vi "test12.1-SyncMessage_Event.vi"(8 "error in (no error)":errorcluster, 11 "TestCase in":refnum<class "testcase-CSMGlobalLog.lvclass">) -> (0 "error out":errorcluster, 3 "TestCase out":refnum<class "testcase-CSMGlobalLog.lvclass">)   [LabVIEW 2017, in "testcase-CSMGlobalLog.lvclass"]
uses:
  testcase-CSMGlobalLog.lvclass
  testcase-CSMGlobalLog.lvclass/testcase-CSMGlobalLog.ctl
  src/user.lib/_NEVSTOP/Communicable State Machine(CSM)/_Support/Typedef/_CSM_GlobalLog_MSG.ctl
  src/user.lib/_NEVSTOP/Communicable State Machine(CSM)/_Support/Typedef/_CSM_Response Source Message.ctl
  src/user.lib/_NEVSTOP/Communicable State Machine(CSM)/_Support/Typedef/_CSM_GlobalLog_MSG_TYPE.ctl
  c0dc643a-0362-49fc-99f4-5251266ba5a0.vi
  src/user.lib/_NEVSTOP/Communicable State Machine(CSM)/_Support/GlobalEvent/GEvt-Generate with Rule Check.vi
  src/user.lib/_NEVSTOP/Communicable State Machine(CSM)/AdvanceAPI/CSM - Convert Error to Argument.vi
  src/user.lib/_NEVSTOP/Communicable State Machine(CSM)/_Support/GlobalEvent/Cache-GEvt Filter Object.vi
  src/user.lib/_NEVSTOP/Communicable State Machine(CSM)/_Support/GlobalEvent/Cache-GEvt Refs.vi
  src/user.lib/_NEVSTOP/Communicable State Machine(CSM)/AdvanceAPI/CSM - Make String Arguments Safe.vi
  src/user.lib/_NEVSTOP/Communicable State Machine(CSM)/_Support/GlobalEvent/GEvt-Convert Filter Rules - v1.2.vi
  src/user.lib/_NEVSTOP/Communicable State Machine(CSM)/_Support/ChangeFlag/FlagInstance-GEvt Filter.vi
  src/user.lib/_NEVSTOP/Communicable State Machine(CSM)/_Support/ChangeFlag/FlagInstance-GEvt Refs.vi
  src/user.lib/_NEVSTOP/Communicable State Machine(CSM)/AdvanceAPI/CSM - Keywords.vi
  src/user.lib/_NEVSTOP/Communicable State Machine(CSM)/_Support/ChangeFlag/ChangeFlag-Read.vi
  src/user.lib/_NEVSTOP/Communicable State Machine(CSM)/_Support/ChangeFlag/ChangeFlagDB.vi
  src/user.lib/_NEVSTOP/Communicable State Machine(CSM)/_Support/GlobalEvent/FGV-GlobalEventRef(lvlibp).vi
  src/user.lib/_NEVSTOP/Communicable State Machine(CSM)/_Support/GlobalEvent/FGV-GlobalEventQueues(lvlibp).vi
  src/user.lib/_NEVSTOP/Communicable State Machine(CSM)/_Support/GlobalEvent/GEvt-Valid Subscribers.vi
  src/user.lib/_NEVSTOP/Communicable State Machine(CSM)/_Support/GlobalEvent/FGV-GEvt Filter Rules(lvlibp).vi
  src/user.lib/_NEVSTOP/Communicable State Machine(CSM)/_Support/GlobalEvent/LogFilter/SettingVIs/Set Global CSM Filter.vi
  src/user.lib/_NEVSTOP/Communicable State Machine(CSM)/_Support/GlobalEvent/LogFilter/SettingVIs/Set Global LogType Filter.vi
  src/user.lib/_NEVSTOP/Communicable State Machine(CSM)/_Support/GlobalEvent/LogFilter/SettingVIs/Set Global State Filter.vi
  src/user.lib/_NEVSTOP/Communicable State Machine(CSM)/_Support/GlobalEvent/LogFilter/SettingVIs/Set Global Broadcast Filter.vi
  src/user.lib/_NEVSTOP/Communicable State Machine(CSM)/_Support/GlobalEvent/LogFilter/SettingVIs/Set Global UserLog Filter.vi
  src/user.lib/_NEVSTOP/Communicable State Machine(CSM)/_Support/GlobalEvent/LogFilter/SettingVIs/Set CSM LogType Filter.vi
  src/user.lib/_NEVSTOP/Communicable State Machine(CSM)/_Support/GlobalEvent/LogFilter/SettingVIs/Set CSM State Filter.vi
  src/user.lib/_NEVSTOP/Communicable State Machine(CSM)/_Support/GlobalEvent/LogFilter/SettingVIs/Set Global StateType Filter.vi
  src/user.lib/_NEVSTOP/Communicable State Machine(CSM)/_Support/GlobalEvent/LogFilter/SettingVIs/Set CSM StateType Filter.vi
  src/user.lib/_NEVSTOP/Communicable State Machine(CSM)/_Support/GlobalEvent/LogFilter/SettingVIs/Set CSM Broadcast Filter.vi
  src/user.lib/_NEVSTOP/Communicable State Machine(CSM)/_Support/GlobalEvent/LogFilter/SettingVIs/Set CSM UserLog Filter.vi
  src/user.lib/_NEVSTOP/Communicable State Machine(CSM)/_Support/GlobalEvent/LogFilter/SettingVIs/Set Periodic Log Filter.vi
  src/user.lib/_NEVSTOP/Communicable State Machine(CSM)/_Support/GlobalEvent/LogFilter/LogFilter - Check.vi
  src/user.lib/_NEVSTOP/Communicable State Machine(CSM)/_Support/GlobalEvent/LogFilter/LogFilter.lvclass
  <vilib>/addons/_JKI Toolkits/VI Tester/TestCase.llb/TestCase.lvclass
  src/user.lib/_NEVSTOP/Communicable State Machine(CSM)/Communicable State Machine.lvlib
  C:/Program Files (x86)/National Instruments/LabVIEW 2017/vi.lib/addons/_JKI Toolkits/VI Tester/TestCase.llb/TestCase.lvclass
panel:
  out "String cache each loop":string
  out "LoopCount":i32
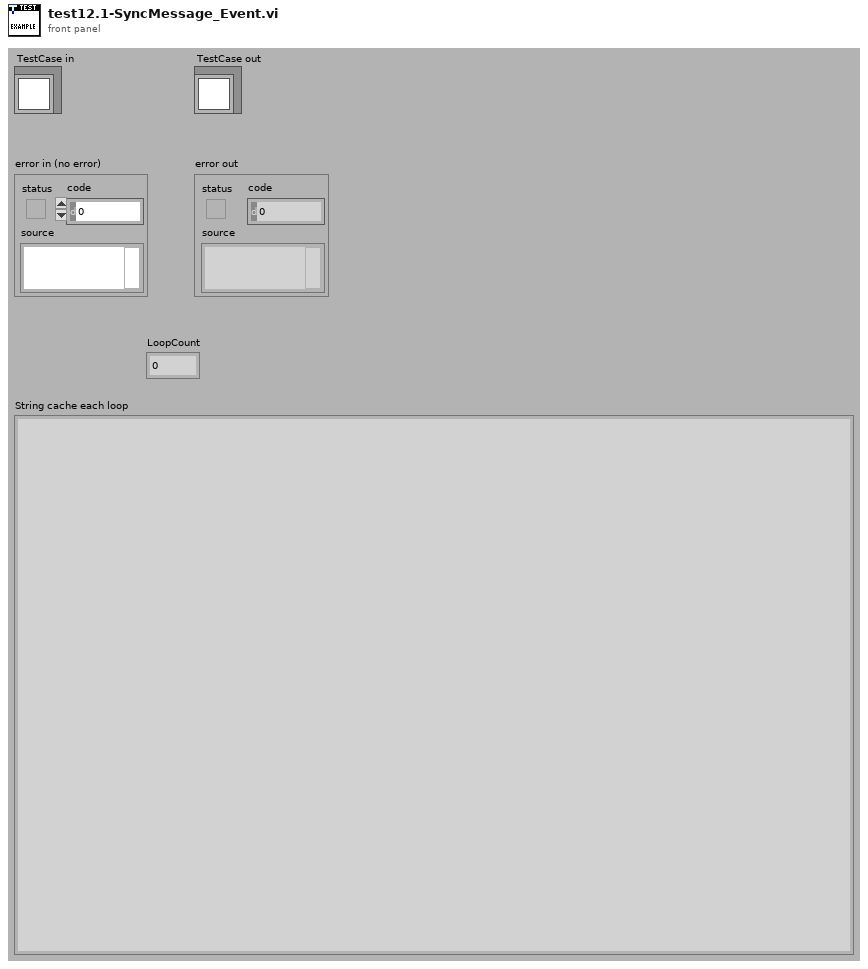
[diagram p1: front panel]
types:
  T1 = typedef "Communicable State Machine.lvlib/_CSM_GlobalLog_MSG.ctl" = cluster{"Name (\"\" to Use UUID)":string, "Current State":string, "Arguments":string, "Source Message":T2, "Source Module":string, "Complete(T)/Start(F)":bool, "LogType":T3, "Time Stamp":timestamp}
  T2 = typedef "Communicable State Machine.lvlib/_CSM_Response Source Message.ctl" = cluster{"‘State":string, "’Arguments":string, "’Error":errorcluster}
  T3 = typedef "Communicable State Machine.lvlib/_CSM_GlobalLog_MSG_TYPE.ctl" = enum16{"User Log", "State Change", "Status", "Interrupt", "Register", "Unregister", "Error Log", "Module Created", "Module Destroyed", "Async Message", "No-Rep Async Message", "Sync Message", "AsyncMsg Complete", "SyncMsg Complete"}
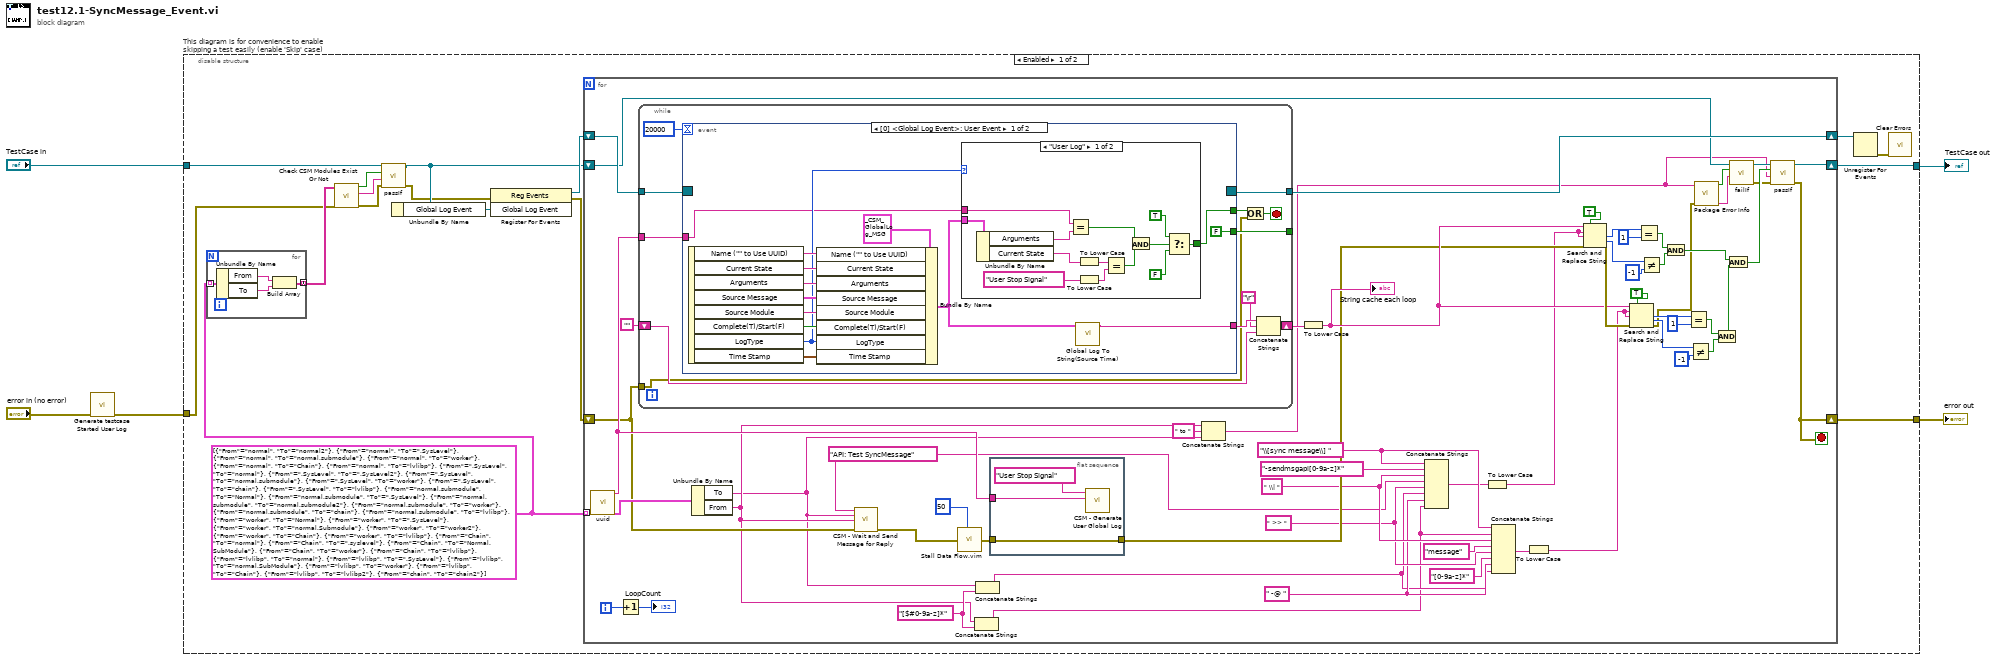
[diagram p0: block diagram]
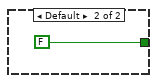
[diagram p2: hidden frame]
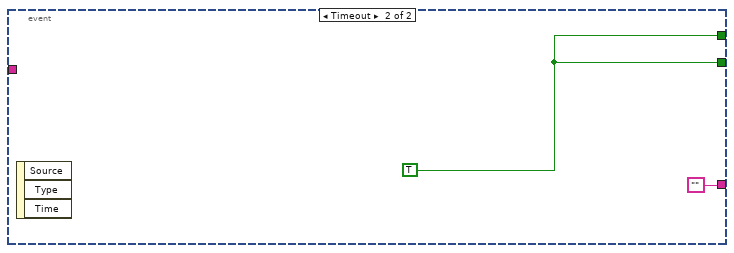
[diagram p3: hidden frame]
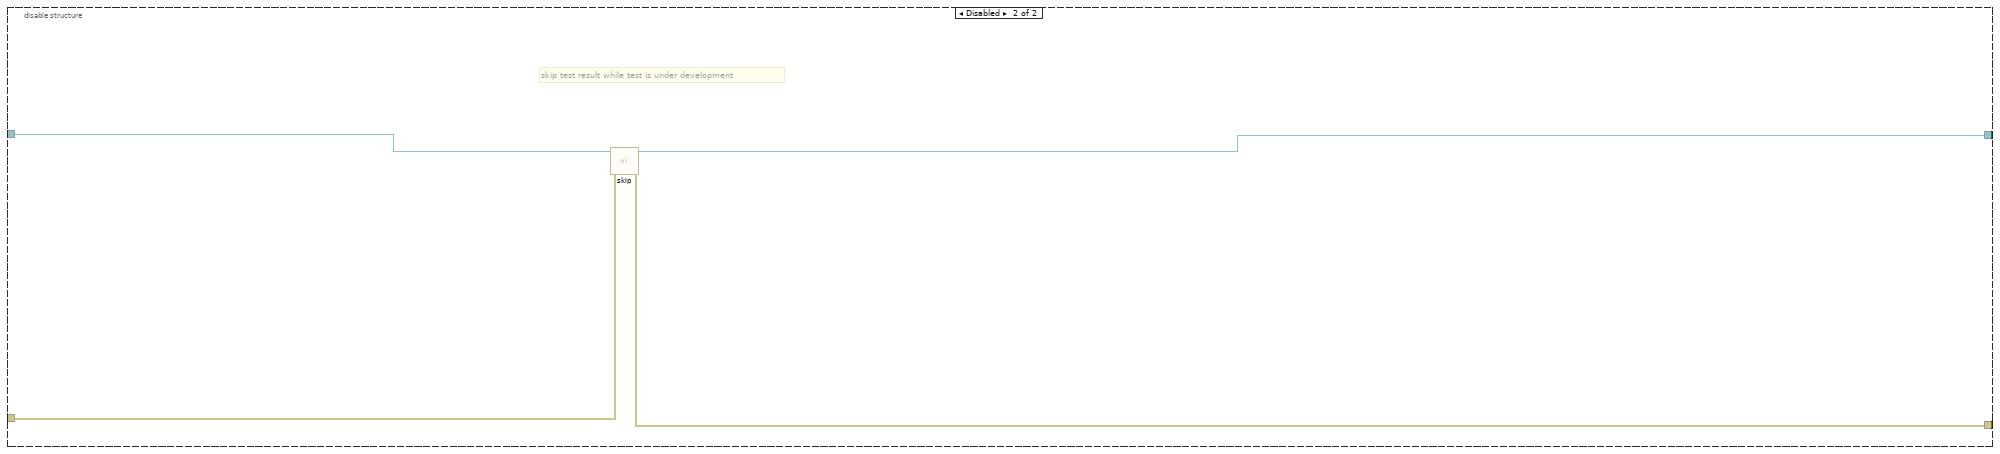
[diagram p4: hidden frame]
diagram:
  n1 = call "Generate testcase Started User Log.vi"("Error In"="error in (no error)") -> ("error out"=w1:errorcluster)  [unwired: 10 in]
  n2 = disable-structure "This diagram is for convenience to enable skipping a test easily (enable 'Skip' case)" shown="Enabled" {
    disable-tunnel: "TestCase in" -> [w9 w133]
    disable-tunnel: [w17 w131] -> w2
    disable-tunnel: [w16 w132] -> w4
    disable-tunnel: w1 -> [w10 w130]
    frame Enabled {
      w11 = cluster{"From":string, "To":string}[] [{"From"="normal", "To"="normal2"}, {"From"="normal", "To"=".SysLevel"}, {"From"="normal", "To"="normal.submodule"}, {"From"="normal", "To"="worker"}, {"From"="normal", "To"="Chain"}, {"From"="normal", "To"="lvlibp"}, {"From"=".SysLevel", "To"="normal"}, {"From"=".SysLevel", "To"=".SysLevel2"}, {"From"=".SysLevel", "To"="normal.submodule"}, {"From"=".SysLevel", "To"="worker"}, {"From"=".SysLevel", "To"="chain"}, {"From"=".SysLevel", "To"="lvlibp"}, {"From"="normal.submodule", "To"="Normal"}, {"From"="normal.submodule", "To"=".SysLevel"}, {"From"="normal.submodule", "To"="normal.submodule2"}, {"From"="normal.submodule", "To"="worker"}, {"From"="normal.submodule", "To"="chain"}, {"From"="normal.submodule", "To"="lvlibp"}, {"From"="worker", "To"="Normal"}, {"From"="worker", "To"=".SysLevel"}, {"From"="worker", "To"="normal.Submodule"}, {"From"="worker", "To"="worker2"}, {"From"="worker", "To"="Chain"}, {"From"="worker", "To"="lvlibp"}, {"From"="Chain", "To"="normal"}, {"From"="Chain", "To"=".syslevel"}, {"From"="Chain", "To"="Normal.SubModule"}, {"From"="Chain", "To"="worker"}, {"From"="Chain", "To"="lvlibp"}, {"From"="lvlibp", "To"="normal"}, {"From"="lvlibp", "To"=".SysLevel"}, {"From"="lvlibp", "To"="normal.SubModule"}, {"From"="lvlibp", "To"="worker"}, {"From"="lvlibp", "To"="Chain"}, {"From"="lvlibp", "To"="lvlibp2"}, {"From"="chain", "To"="chain2"}]
      n3 = for {
        tunnel: w11 -> [w25] mode=indexing
        tunnel: [w22] -> w13 mode=concatenating
        n4 = Unbundle By Name(w25) -> ("From"=w24:string, "To"=w23:string)
        n5 = Build Array(w24, w23) -> (w22:string[])
      }
      n6 = call "Check CSM Modules Exist Or Not.vi"("error in"=w10, "CSM names in"=w13) -> ("error out"=w15:errorcluster, "Debug string"=w14:string, "All Modules Exist?"=w12:bool)  [unwired: 7 in]
      n7 = call-dynamic "passIf.vi"("error in (no error)"=w15, "message (\"\")"=w14, "pass"=w12, "TestCase in"=w9) -> ("error out"=w7:errorcluster, "TestCase out"=w8:refnum<class "testcase-CSMGlobalLog.lvclass">)  [unwired: 6 in]
      n8 = Unbundle By Name(w8) -> ("Global Log Event"=w21:refnum<user-event>)
      n9 = register-events(error in=w7, w21) -> (reference out=w20:refnum<event-registration>, error out=w18:errorcluster)  [unwired: 1 in]
      n10 = for {
        shift-right: [w83] -> w19
        shift-left: w20 -> [w84]
        shift-right: [w80] -> w16
        shift-left: w18 -> [w36]
        tunnel: w11 -> [w61] mode=indexing
        shift-right: [w82] -> w17
        shift-left: w8 -> [w34]
        i -> [w58]
        stop <- w80 stop-if-true
        w39 = "[$#0-9a-z]*" ("string")
        w45 = " -@ "
        w47 = " >> "
        w49 = " \\| "
        w50 = "\\[sync message\\] "
        w42 = "API: Test SyncMessage" ("State")
        n11 = call "uuid.vi"() -> ("UUID"=w59:string)  [unwired: 11 in]
        n12 = Increment(x=w58) -> (x+1=→"LoopCount":i32)
        n13 = while {
          tunnel: w84 -> [w99]
          tunnel: [w98] -> w83
          shift-right: [w91] -> w52
          shift-left: "" -> [w94]
          tunnel: w59 -> [w96]
          tunnel: [w95] -> _
          tunnel: w36 -> [w88]
          stop <- w90 stop-if-true
          n14 = event shown="[0] <Global Log Event>: User Event" {
            selector: w99 -> [_ _]
            dyn-events: [_ _] -> w98
            timeout: 20000 -> [_ _]
            tunnel: [w100 ""] -> w93
            tunnel: [w102 w129] -> w89
            tunnel: w96 -> [w103 _]
            tunnel: [FALSE ("Stop") w129] -> w95
            event User Event {
              n15 = event-data() -> ("Name (\"\" to Use UUID)"=w112:string, "Current State"=w111:string, "Arguments"=w110:string, "Source Message"=w109:T2, "Source Module"=w108:string, "Complete(T)/Start(F)"=w107:bool, "LogType"=w104:T3, "Time Stamp"=w106:timestamp)  [unwired: 1 in]
              n16 = Bundle By Name(cluster=T1 {"Name (\"\" to Use UUID)"="", "Current State"="", "Arguments"="", "Source Message"={"‘State"="", "’Arguments"="", "’Error"={"status"=FALSE, "code"=0, "source"=""}}, "Source Module"="", "Complete(T)/Start(F)"=FALSE, "LogType"=enum."State Change", "Time Stamp"=timestamp(0 s since 1904-01-01)} ("Cross CSM Data"), "Name (\"\" to Use UUID)"=w112, "Current State"=w111, "Arguments"=w110, "Source Message"=w109, "Source Module"=w108, "Complete(T)/Start(F)"=w107, "LogType"=w104, "Time Stamp"=w106) -> (w101:T1)
              n17 = case shown="\"User Log\"" w104 {
                tunnel: w101 -> [w126 _]
                tunnel: w103 -> [w125 _]
                tunnel: [w114 FALSE] -> w102
                frame "User Log" {
                  n18 = Unbundle By Name(w126) -> ("Arguments"=w124:string, "Current State"=w123:string)
                  n19 = Equal?(x=w125, y=w124) -> (x = y?=w118:bool)
                  n20 = To Lower Case(string=w123) -> (all lower case string=w122:string)
                  n21 = To Lower Case(string="User Stop Signal" ("Log")) -> (all lower case string=w120:string)
                  n22 = Equal?(x=w122, y=w120) -> (x = y?=w119:bool)
                  n23 = And(x=w118, y=w119) -> (x .and. y?=w117:bool)
                  n24 = Select(t=TRUE, s=w117, f=FALSE) -> (s? t:f=w114:bool)
                }
                frame Default {
                }
              }
              n25 = call "Global Log To String(Source Time).vi"("Log"=w101) -> ("Log String"=w100:string)  [unwired: 9 in]
            }
            event Timeout {
              w129 = TRUE ("Stop")
              n26 = event-data() -> ()  [unwired: 1 in, 3 out]
            }
          }
          n27 = Or(x=w89, y=w88) -> (x .or. y?=w90:bool)
          n28 = Concatenate Strings(w93, "\r", w94) -> (w91:string)
        }
        n29 = Unbundle By Name(w61) -> ("To"=w28:string, "From"=w29:string)
        n30 = call "CSM - Wait and Send Message for Reply.vi"("State"=w42, "Arguments (\"\")"=w28, "Target Module"=w29, "Error In (No Error)"=w36) -> ("error out"=w55:errorcluster)  [unwired: 8 in, 3 out]
        n31 = call "Stall Data Flow.vim"("value in"=w55, "milliseconds to wait"=u32 50) -> ("value out"=w60:errorcluster)  [unwired: 1 out]
        n32 = Concatenate Strings(w29, w39) -> (w37:string)
        n33 = Concatenate Strings(w28, w39) -> (w38:string)
        n34 = flat-sequence {
          tunnel: w59 -> [w86]
          tunnel: w60 -> [w85]
          tunnel: [w85] -> w53
          frame #0 {
            n35 = call "CSM - Generate User Global Log.vi"("Arguments"=w86, "Log"="User Stop Signal") -> ()  [unwired: 9 in, 1 out]
          }
        }
        n36 = Concatenate Strings(w29, " to " ("string"), w28) -> (w26:string)
        n37 = To Lower Case(string=w52) -> (all lower case string=w54:string)
        "String cache each loop" <- w54
        n38 = Concatenate Strings(w50, "-sendmsgapi[0-9a-z]*", w49, w42, w47, w38, w45, w37) -> (w44:string)
        n39 = To Lower Case(string=w44) -> (all lower case string=w41:string)
        n40 = Concatenate Strings(w50, w37, w49, "message", w47, "[0-9a-z]*", w45, w38) -> (w43:string)
        n41 = To Lower Case(string=w43) -> (all lower case string=w40:string)
        n42 = Search and Replace String(replace all?=TRUE ("replace all? (F)"), input string=w54, search string=w41, replace string=w41, error in=w53) -> (number of replacements=w69:i32, offset past replacement=w70:i32, error out=w77:errorcluster)  [unwired: 3 in, 1 out]
        n43 = Search and Replace String(replace all?=TRUE ("replace all? (F)"), input string=w54, search string=w40, replace string=w40, error in=w77) -> (number of replacements=w76:i32, offset past replacement=w75:i32, error out=w30:errorcluster)  [unwired: 3 in, 1 out]
        n44 = Equal?(x=w69, y=1) -> (x = y?=w71:bool)
        n45 = Not Equal?(x=w70, y=-1) -> (x != y?=w72:bool)
        n46 = And(x=w71, y=w72) -> (x .and. y?=w79:bool)
        n47 = Equal?(x=w76, y=1) -> (x = y?=w74:bool)
        n48 = Not Equal?(x=w75, y=-1) -> (x != y?=w73:bool)
        n49 = call "Package Error Info.vi"("error in"=w30, "String in"=w26) -> ("packed error info out"=w31:string, "error status"=w35:bool)  [unwired: 8 in]
        n50 = And(x=w74, y=w73) -> (x .and. y?=w78:bool)
        n51 = And(x=w79, y=w78) -> (x .and. y?=w57:bool)
        n52 = call-dynamic "failIf.vi"("message (\"\")"=w31, "fail"=w35, "TestCase in"=w34) -> ("error out"=w32:errorcluster, "TestCase out"=w33:refnum<class "testcase-CSMGlobalLog.lvclass">)  [unwired: 7 in]
        n53 = call-dynamic "passIf.vi"("error in (no error)"=w32, "message (\"\")"=w26, "pass"=w57, "TestCase in"=w33) -> ("error out"=w80:errorcluster, "TestCase out"=w82:refnum<class "testcase-CSMGlobalLog.lvclass">)  [unwired: 6 in]
      }
      n54 = Unregister For Events(event registration refnum=w19) -> (error out=w6:errorcluster)  [unwired: 1 in]
      n55 = call <vilib>:"Clear Errors.vi"("error in (no error)"=w6) -> ()  [unwired: 5 in, 2 out]
    }
    frame Disabled {
      # "skip test result while test is under development"
      n56 = call <vilib>:"skip.vi"("error in (no error)"=w130, "TestCase in"=w133) -> ("error out"=w132:errorcluster, "TestCase out"=w131:refnum<class "testcase-CSMGlobalLog.lvclass">)  [unwired: 8 in]
    }
  }
  "error out" <- w4
  "TestCase out" <- w2
